vi "Langmuir Probe.vi"() -> ()   [LabVIEW 2016]
uses:
  <vilib>/Analysis/baseanly.llb/Mean (DBL).vi
  <vilib>/Analysis/NI_AALBase.lvlib
panel:
  out "Ln Plot":cluster{"Y":dbl[], "Y":dbl[]}(graph)
  in  "Values":dbl[](array[numeric])
  in  "Operating Conditions":string[](array[string])=["Time [s]", "Time [hr]", "Current Voltage [V]", "Langmuir Current [A]", "Langmuir Voltage [V]"]
  out "Voltage Setting":dbl
  in  "Stop Voltage":i32
  in  "Start Voltage":i32
  out "Langmuir Voltage [V]":dbl
  in  "Resistance [Ohm]":dbl
  out "XY Graph":cluster{"Y":dbl[], "Y":dbl[]}(graph)
  in  "Plot Button":bool
  in  "Test Operator":string
  out "Langmuir Current [A]":dbl
  out "Current Voltage [V]":dbl
  out "Elapsed Time [hr]":dbl
  out "Elapsed Time [s]":dbl
  out "Err":bool
  in  "error in":errorcluster
  out "error out":errorcluster
  in  "stop":bool
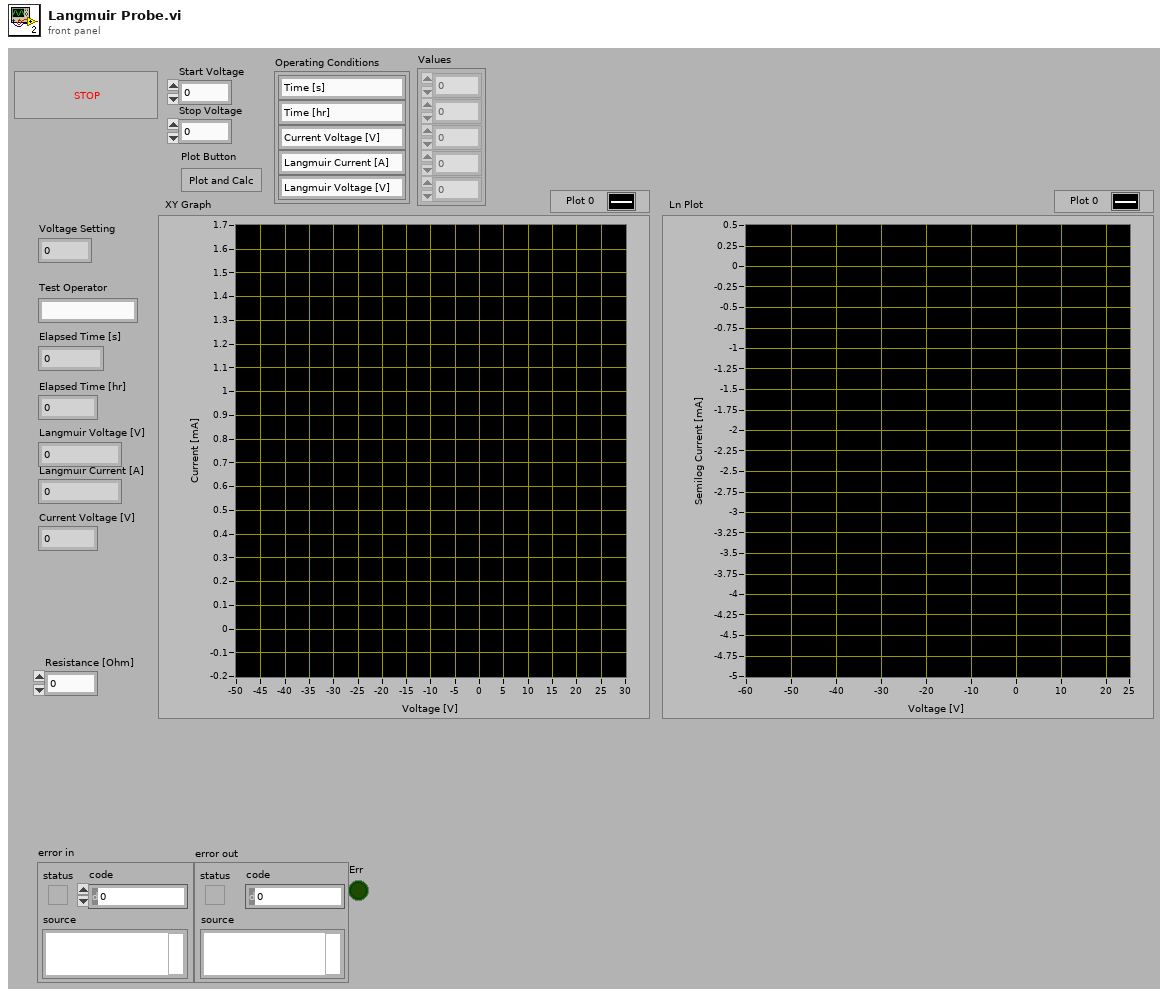
[diagram p1: front panel]
types:
  T1 = enum16{"open", "open or create", "create or replace", "create", "open (read-only)"}
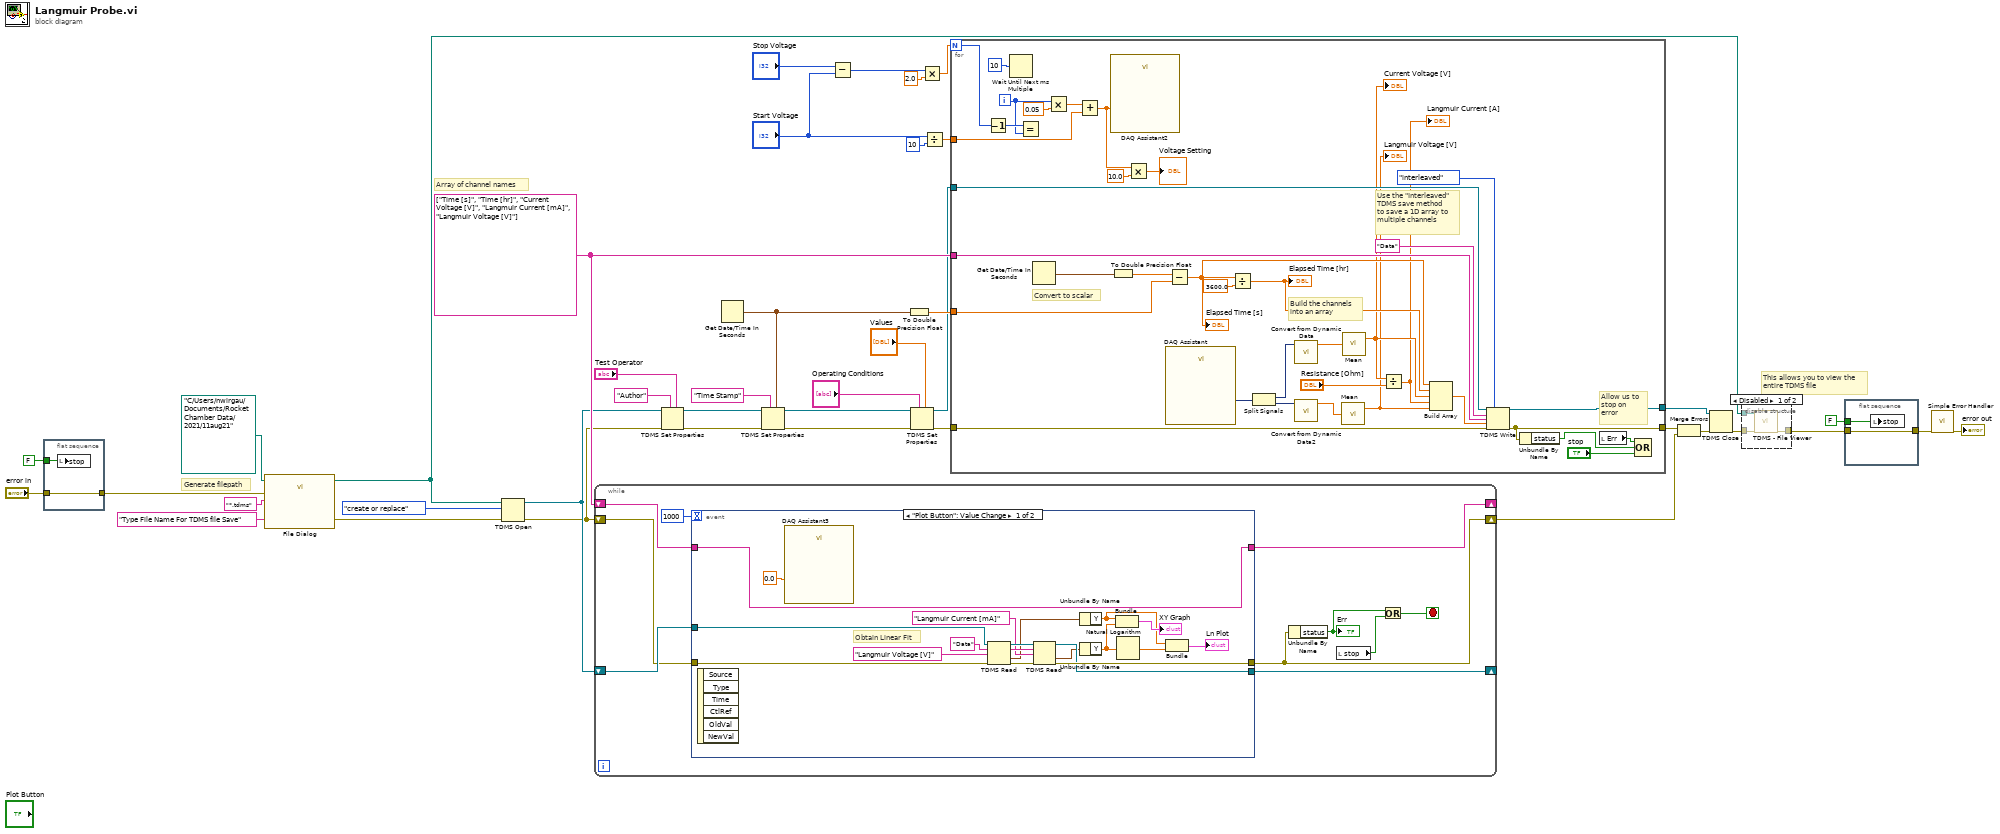
[diagram p0: block diagram]
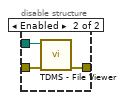
[diagram p2: hidden frame]
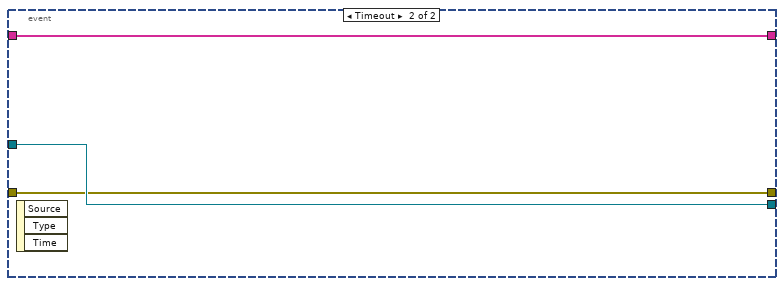
[diagram p3: hidden frame]
diagram:
  w29 = string[] ["Time [s]", "Time [hr]", "Current Voltage [V]", "Langmuir Current [mA]", "Langmuir Voltage [V]"] ("channel name(s) in (Untitled)")
  # "This allows you to view the\nentire TDMS file"
  # "Generate filepath"
  # "Array of channel names"
  n1 = flat-sequence {
    tunnel: "error in" -> [w43]
    tunnel: [w43] -> w27
    tunnel: FALSE ("stop") -> [w42]
    frame #0 {
      n2 = local write "stop"(w42) -> ()
    }
  }
  n3 = call "File Dialog"("start path"=path "C:/Users/nwirgau/Documents/Rocket Chamber Data/2021/11aug21", "prompt"="Type File Name For TDMS file Save", "error in"=w27, "pattern (all files)"="*.tdms") -> ("selected path"=w26:path, "error out"=w25:errorcluster)  [unwired: 8 in, 2 out]
  n4 = TDMS Open(8:w25, 10:T1."create or replace" ("operation (0:open)"), 11:w26) -> (0:w15:errorcluster, 3:w22:refnum<k34>)  [unwired: 4 in]
  n5 = while {
    shift-right: [w47] -> w33
    shift-left: w15 -> [w52]
    shift-right: [w51] -> _
    shift-left: w22 -> [w53]
    shift-right: [w49] -> _
    shift-left: w29 -> [w50]
    stop <- w46 stop-if-true
    n6 = event shown="[0] \"Plot Button\": Value Change" {
      selector: _ -> [_ _]
      dyn-events: _ -> [_ _]
      timeout: 1000 -> [_ _]
      tunnel: w53 -> [w72 w75]
      tunnel: w52 -> [w71 w73]
      tunnel: [w62 w73] -> w47
      tunnel: [w61 w75] -> w51
      tunnel: w50 -> [w60 w74]
      tunnel: [w60 w74] -> w49
      event "Plot Button": Value Change {
        # "Obtain Linear Fit"
        n7 = event-data() -> ()  [unwired: 1 in, 6 out]
        n8 = call "DAQ Assistant3"("data"=0.0 ("t")) -> ()  [unwired: 17 in, 2 out]
        n9 = TDMS Read(0:w72, 5:"Data" ("group name in"), 7:"Langmuir Voltage [V]" ("group name in"), 11:w71) -> (4:w68:refnum<k34>, 6:w67:string, 10:w64:waveform(dbl), 15:w66:errorcluster)  [unwired: 4 in, 2 out]
        n10 = TDMS Read(0:w68, 5:w67, 7:"Langmuir Current [mA]" ("group name in"), 11:w66) -> (4:w61:refnum<k34>, 10:w58:waveform(dbl), 15:w62:errorcluster)  [unwired: 4 in, 3 out]
        n11 = Unbundle By Name(w64) -> ("Y"=w55:dbl[])
        n12 = Unbundle By Name(w58) -> ("Y"=w57:dbl[])
        n13 = Bundle("Y"=w55, "Y"=w57) -> (→"XY Graph":cluster{"Y":dbl[], "Y":dbl[]})  [unwired: 1 in]
        n14 = Natural Logarithm(1:w57) -> (0:w56:dbl[])
        n15 = Bundle("Y"=w55, w56) -> (→"Ln Plot":cluster{"Y":dbl[], dbl[]})  [unwired: 1 in]
      }
      event Timeout {
        n16 = event-data() -> ()  [unwired: 1 in, 3 out]
      }
    }
    n17 = Unbundle By Name(w47) -> ("status"=w45:bool)
    "Err" <- w45
    n18 = local read "stop"() -> (w48:bool)
    n19 = Or(x=w45, y=w48) -> (x .or. y?=w46:bool)
  }
  n20 = TDMS Set Properties(5:"Test Operator", 7:"Author", 8:w15, 11:w22) -> (0:w23:errorcluster, 3:w21:refnum<k34>)  [unwired: 2 in, 2 out]
  n21 = Get Date/Time In Seconds() -> (seconds since 1Jan1904=w17:timestamp)
  n22 = TDMS Set Properties(5:w17, 7:"Time Stamp", 8:w23, 11:w21) -> (0:w6:errorcluster, 3:w5:refnum<k34>)  [unwired: 2 in, 2 out]
  n23 = Subtract(x="Stop Voltage", y="Start Voltage") -> (x-y=w13:i32)
  n24 = To Double Precision Float(number=w17) -> (double precision float=w28:dbl)
  n25 = TDMS Set Properties(5:"Values", 7:"Operating Conditions", 8:w6, 11:w5) -> (0:w2:errorcluster, 3:w1:refnum<k34>)  [unwired: 2 in, 2 out]
  n26 = Multiply(x=w13, y=2.0) -> (x*y=w8:dbl)
  n27 = Divide(x="Start Voltage", y=10) -> (x/y=w7:dbl)
  n28 = for {
    N: w8 -> [w82]
    tunnel: w1 -> [w97]
    tunnel: [w111] -> w41
    tunnel: [w107] -> w34
    tunnel: w2 -> [w98]
    tunnel: w29 -> [w108]
    tunnel: w28 -> [w102]
    tunnel: w7 -> [w80]
    i -> [w81]
    # "Allow us to \nstop on \nerror"
    # "Use the \"Interleaved\"\nTDMS save method\nto save a 1D array to\nmultiple channels"
    # "Build the channels\ninto an array"
    # "Convert to scalar"
    n29 = Decrement(x=w82) -> (x-1=w84:i32)
    n30 = Wait Until Next ms Multiple(millisecond multiple=u32 10) -> ()  [unwired: 1 out]
    n31 = Equal?(x=w84, y=w81) -> ()  [unwired: 1 out]
    n32 = Get Date/Time In Seconds() -> (seconds since 1Jan1904=w103:timestamp)
    n33 = Multiply(x=w81, y=0.05) -> (x*y=w83:dbl)
    n34 = Add(x=w83, y=w80) -> (x+y=w78:dbl)
    n35 = call "DAQ Assistant2"("data"=w78) -> ()  [unwired: 17 in, 2 out]
    n36 = To Double Precision Float(number=w103) -> (double precision float=w101:dbl)
    n37 = Multiply(x=w78, y=10.0) -> (x*y=→"Voltage Setting":dbl)
    n38 = call "DAQ Assistant"() -> ("data"=w90:dynamicdata)  [unwired: 17 in, 2 out]
    n39 = Subtract(x=w101, y=w102) -> (x-y=w100:dbl)
    "Elapsed Time [s]" <- w100
    n40 = Divide(x=w100, y=3600.0) -> (x/y=w96:dbl)
    "Elapsed Time [hr]" <- w96
    n41 = Split Signals(w90) -> (w89:dynamicdata, w88:dynamicdata)  [unwired: 2 in]
    n42 = call "Convert from Dynamic Data"("Dynamic Data Type"=w89) -> ("Array"=w94:dbl[])  [unwired: 3 in]
    n43 = call "Convert from Dynamic Data2"("Dynamic Data Type"=w88) -> ("Array"=w87:dbl[])  [unwired: 3 in]
    n44 = call-poly <vilib>:"Mean.vi"("X"=w87) -> ("mean"=w86:dbl)  [unwired: 1 out]
    "Langmuir Voltage [V]" <- w86
    n45 = call-poly <vilib>:"Mean.vi"("X"=w94) -> ("mean"=w93:dbl)  [unwired: 1 out]
    "Current Voltage [V]" <- w93
    n46 = Divide(x=w93, y="Resistance [Ohm]") -> (x/y=w92:dbl)
    "Langmuir Current [A]" <- w92
    n47 = Build Array(w100, w96, w93, w92, w86) -> (w109:dbl[])
    n48 = TDMS Write(0:w97, 1:enum16{"decimated", "interleaved"}."interleaved" ("data layout (0:decimated)"), 5:"Data" ("group name in (Untitled)"), 7:w108, 9:w109, 11:w98) -> (4:w111:refnum<k34>, 15:w107:errorcluster)  [unwired: 2 out]
    n49 = Unbundle By Name(w107) -> ("status"=w106:bool)
    n50 = local read "Err"() -> (w104:bool)
    n51 = Compound Arithmetic op=OR(w104, w106, "stop") -> ()  [unwired: 1 out]
  }
  n52 = Merge Errors(w34, w33) -> (w32:errorcluster)
  n53 = TDMS Close(8:w32, 11:w41) -> (0:w40:errorcluster)  [unwired: 1 out]
  n54 = disable-structure shown="Disabled" {
    disable-tunnel: w40 -> [w114 w117]
    disable-tunnel: w26 -> [w113 w115]
    disable-tunnel: [w112 w116] -> w35
    frame Disabled {
      n55 = call <vilib>:"TDMS - File Viewer.vi"("error in (no error)"=w114, "file path"=w113) -> ("error out"=w112:errorcluster)  [unwired: 4 in, 1 out]
    }
    frame Enabled {
      n56 = call <vilib>:"TDMS - File Viewer.vi"("error in (no error)"=w117, "file path"=w115) -> ("error out"=w116:errorcluster)  [unwired: 4 in, 1 out]
    }
  }
  n57 = flat-sequence {
    tunnel: w35 -> [w119]
    tunnel: [w119] -> w31
    tunnel: FALSE ("stop") -> [w118]
    frame #0 {
      n58 = local write "stop"(w118) -> ()
    }
  }
  n59 = call <vilib>:"Simple Error Handler.vi"("error in (no error)"=w31) -> ("error out"=→"error out":errorcluster)  [unwired: 4 in, 4 out]
